vi "Variant Type Desc To Element.vi"(9 "Data String":string, 10 "Type Descriptor":i16[](array[numeric])) -> (3 "Variant List":T1)   [LabVIEW 2011, in "JSON Scalar.lvclass"]
doc: "Retrieves the name and data type from the type descriptor"
uses:
  JSON Scalar.lvclass
  Variant Data Typdef.ctl
  <vilib>/Utility/VariantDataType/Type.ctl
  <vilib>/Utility/VariantDataType/VariantType.lvlib
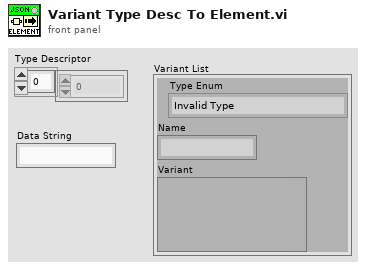
[diagram p1: front panel]
types:
  T1 = typedef "JSON Scalar.lvclass/Variant Data Typdef.ctl" = cluster{"Type Enum":T2, "Name":string, "Variant":variant}
  T2 = typedef "VariantType.lvlib/Type.ctl" = enum8{"Invalid Type", "Void", "I8", "I16", "I32", "I64", "U8", "U16", "U32", "U64", "Single Float", "Double Float", "Extended Float", "Single Complex", "Double Complex", "Extended Complex", "Enum U8", "Enum U16", "Enum U32", "Enum U64", "Single Float With Unit", "Double Float With Unit", "Extended Float With Unit", "Single Complex with Unit", "Double Complex with Unit", "Extended Complex with Unit", "Boolean", "String", "Path", "Picture", "Tag", "Array", "Cluster", "Variant", "LV Variant", "Waveform", "Timestamp", "Digital Waveform", "Digital Data", "ExpressData", "Refnum", "External Data", "VI", "Poly VI", "LabVIEW Class Instance", "Fixed Point"}
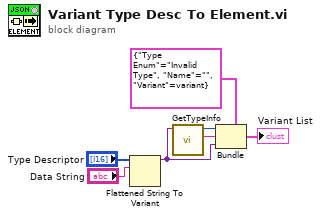
[diagram p0: block diagram]
diagram:
  n1 = Flattened String To Variant(6:"Data String", 7:"Type Descriptor") -> (3:w4:variant)  [unwired: 1 in, 1 out]
  n2 = call <vilib>:"GetTypeInfo.vi"("Variant"=w4) -> ("Name"=w6:string, "Type Enum"=w5:T2)  [unwired: 6 in, 3 out]
  n3 = Bundle(cluster=T1 {"Type Enum"=enum."Invalid Type", "Name"="", "Variant"=variant} ("cluster in"), "Type Enum"=w5, "Name"=w6, "Variant"=w4) -> (→"Variant List":T1)
